vi "LSX Set BPZ Trackball Back Lash.vi"(6 "dR":dbl, 7 "dZ":dbl, 8 "error in (no error)":errorcluster, 9 "dY":dbl, 10 "dX":dbl, 11 "lLSID":i32) -> (0 "error out":errorcluster, 3 "function return":i32)   [LabVIEW 2016, in "Tango_DLL.lvlib"]
doc: "TANGOAPI int TANGOCALL LSX_SetBPZTrackballBackLash (int lLSID, double dX, double dY, double dZ, double dR);"
uses:
  Tango_DLL.lvlib
  2017/Microscope Control/Device Library/Stages/Marzhauser/SCAN IM 120 x 80/Tango DLL VIs/Tango_DLL.dll
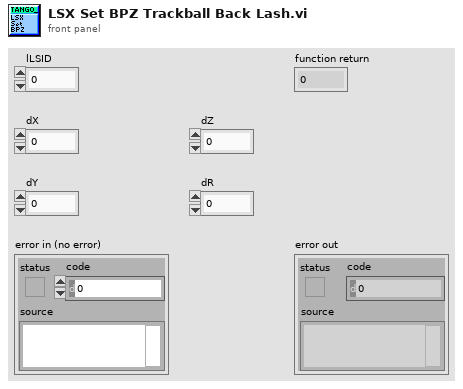
[diagram p1: front panel]
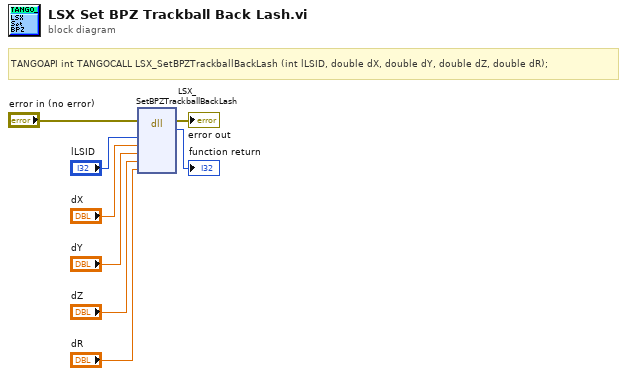
[diagram p0: block diagram]
diagram:
  # "TANGOAPI int TANGOCALL LSX_SetBPZTrackballBackLash (int lLSID, double dX, double dY, double dZ, double dR);"
  n1 = dll-call lib="C:/Users/4PiSMS/Documents/Microscope Control/2017/Microscope Control/Device Library/Stages/Marzhauser/SCAN IM 120 x 80/Tango DLL VIs/Tango_DLL.*" fn="LSX_SetBPZTrackballBackLash"(error in="error in (no error)", "lLSID"="lLSID", "dX"="dX", "dY"="dY", "dZ"="dZ", "dR"="dR") -> (error out=→"error out":errorcluster, →"function return":i32)  [unwired: 7 in, 1 out]
